vi "Colores_c.vi"() -> ()   [LabVIEW 2017]
panel:
  out "Verde 3":u32[](array[colorbox])
  out "Verde 2":u32[](array[colorbox])
  out "Azul":u32[](array[colorbox])
  out "Verde":u32[](array[colorbox])
  out "Rojo":u32[](array[colorbox])
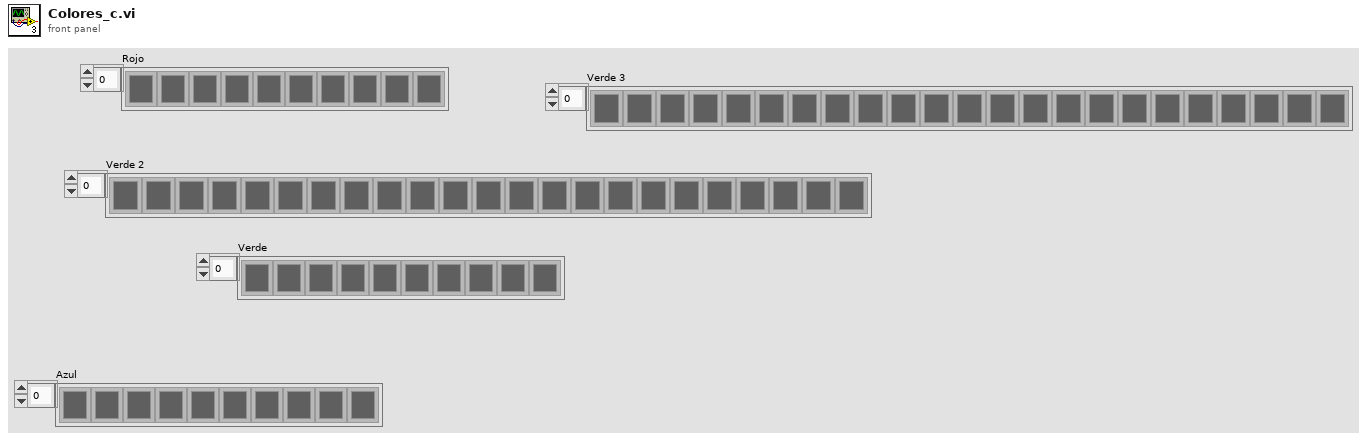
[diagram p1: front panel]
types:
  T1 = typedef "Semaphore RefNum" = refnum<k1>
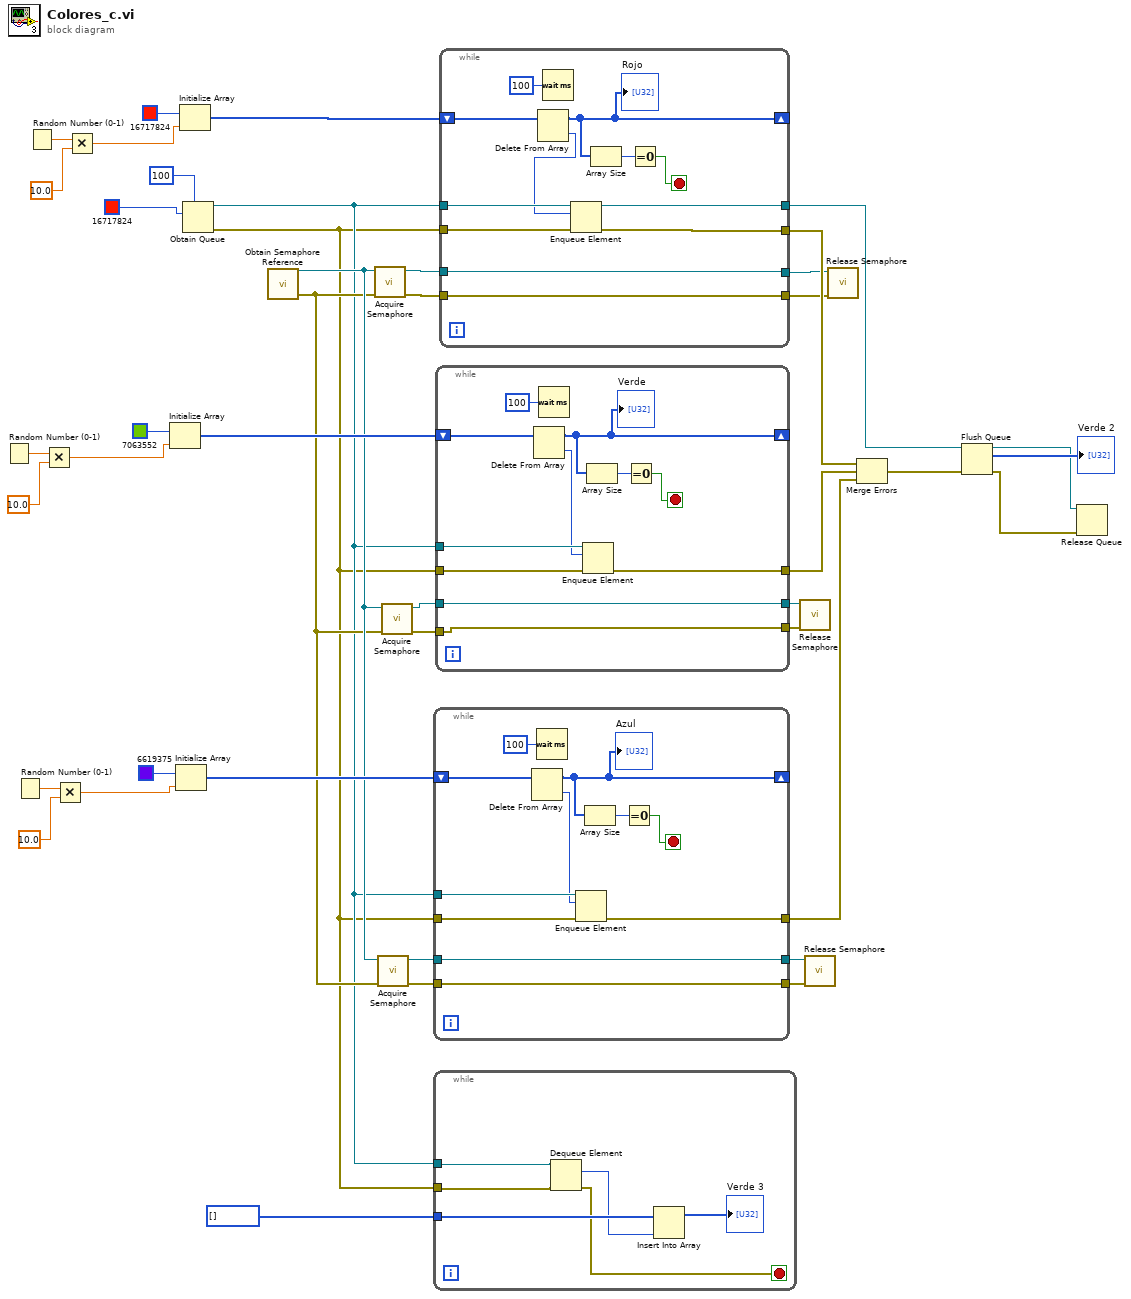
[diagram p0: block diagram]
diagram:
  n1 = Random Number (0-1)() -> (number: 0 to 1=w40:dbl)
  n2 = Random Number (0-1)() -> (number: 0 to 1=w38:dbl)
  n3 = Random Number (0-1)() -> (number: 0 to 1=w42:dbl)
  n4 = Multiply(x=w40, y=10.0) -> (x*y=w32:dbl)
  n5 = Multiply(x=w38, y=10.0) -> (x*y=w33:dbl)
  n6 = Multiply(x=w42, y=10.0) -> (x*y=w31:dbl)
  n7 = Initialize Array "Initialize Array"(u32 7063552, w32) -> (w28:u32[])
  n8 = Initialize Array "Initialize Array"(u32 6619375, w33) -> (w29:u32[])
  n9 = Initialize Array "Initialize Array"(u32 16717824, w31) -> (w30:u32[])
  n10 = Obtain Queue(max queue size (-1, unlimited)=100, element data type=u32 16717824) -> (queue out=w6:refnum<queue>, error out=w5:errorcluster)  [unwired: 3 in, 1 out]
  n11 = call <vilib>:"Obtain Semaphore Reference.vi"() -> ("error out"=w15:errorcluster, "semaphore"=w16:T1)  [unwired: 5 in, 1 out]
  n12 = call <vilib>:"Acquire Semaphore.vi"("error in (no error)"=w15, "semaphore"=w16) -> ("error out"=w18:errorcluster, "semaphore out"=w19:T1)  [unwired: 3 in, 1 out]
  n13 = call <vilib>:"Acquire Semaphore.vi"("error in (no error)"=w15, "semaphore"=w16) -> ("error out"=w12:errorcluster, "semaphore out"=w14:T1)  [unwired: 3 in, 1 out]
  n14 = call <vilib>:"Acquire Semaphore.vi"("error in (no error)"=w15, "semaphore"=w16) -> ("error out"=w10:errorcluster, "semaphore out"=w7:T1)  [unwired: 3 in, 1 out]
  n15 = while {
    shift-right: [w50] -> _
    shift-left: w29 -> [w53]
    tunnel: w6 -> [w48]
    tunnel: w5 -> [w47]
    tunnel: [w46] -> w23
    tunnel: w14 -> [w44]
    tunnel: [w44] -> w13
    tunnel: w12 -> [w43]
    tunnel: [w43] -> w11
    stop <- w51 stop-if-true
    n16 = Delete From Array(array=w53) -> (deleted portion=w45:u32, array with subset deleted=w50:u32[])  [unwired: 2 in]
    "Azul" <- w50
    n17 = Wait (ms)(milliseconds to wait=u32 100) -> ()  [unwired: 1 out]
    n18 = Enqueue Element(queue=w48, element=w45, error in (no error)=w47) -> (error out=w46:errorcluster)  [unwired: 1 in, 2 out]
    n19 = Array Size(array=w50) -> (size(s)=w52:i32)
    n20 = Equal To 0?(x=w52) -> (x = 0?=w51:bool)
  }
  n21 = while {
    tunnel: w6 -> [w58]
    tunnel: w5 -> [w57]
    tunnel: u32[] [] -> [w59]
    stop <- w56 stop-if-true
    n22 = Dequeue Element(queue=w58, error in (no error)=w57) -> (element=w55:u32, error out=w56:errorcluster)  [unwired: 1 in, 2 out]
    n23 = Insert Into Array(array=w59, new element=w55) -> (→"Verde 3":u32[])  [unwired: 1 in]
  }
  n24 = while {
    shift-right: [w67] -> _
    shift-left: w28 -> [w70]
    tunnel: w6 -> [w65]
    tunnel: w5 -> [w64]
    tunnel: [w63] -> w24
    tunnel: w10 -> [w61]
    tunnel: [w61] -> w9
    tunnel: [w60] -> w8
    tunnel: w7 -> [w60]
    stop <- w68 stop-if-true
    n25 = Delete From Array(array=w70) -> (deleted portion=w62:u32, array with subset deleted=w67:u32[])  [unwired: 2 in]
    "Verde" <- w67
    n26 = Wait (ms)(milliseconds to wait=u32 100) -> ()  [unwired: 1 out]
    n27 = Enqueue Element(queue=w65, element=w62, error in (no error)=w64) -> (error out=w63:errorcluster)  [unwired: 1 in, 2 out]
    n28 = Array Size(array=w67) -> (size(s)=w69:i32)
    n29 = Equal To 0?(x=w69) -> (x = 0?=w68:bool)
  }
  n30 = while {
    shift-right: [w79] -> _
    shift-left: w30 -> [w82]
    tunnel: w6 -> [w77]
    tunnel: w5 -> [w75]
    tunnel: [w74] -> w25
    tunnel: [w73] -> w22
    tunnel: [w72] -> w20
    tunnel: w19 -> [w72]
    tunnel: w18 -> [w71]
    tunnel: [w71] -> w17
    stop <- w80 stop-if-true
    n31 = Delete From Array(array=w82) -> (deleted portion=w76:u32, array with subset deleted=w79:u32[])  [unwired: 2 in]
    "Rojo" <- w79
    n32 = Wait (ms)(milliseconds to wait=u32 100) -> ()  [unwired: 1 out]
    n33 = Enqueue Element(queue=w77, element=w76, error in (no error)=w75) -> (queue out=w73:refnum<queue>, error out=w74:errorcluster)  [unwired: 1 in, 1 out]
    n34 = Array Size(array=w79) -> (size(s)=w81:i32)
    n35 = Equal To 0?(x=w81) -> (x = 0?=w80:bool)
  }
  n36 = call <vilib>:"Release Semaphore.vi"("error in (no error)"=w9, "semaphore"=w8) -> ()  [unwired: 4 in, 2 out]
  n37 = call <vilib>:"Release Semaphore.vi"("error in (no error)"=w11, "semaphore"=w13) -> ()  [unwired: 4 in, 2 out]
  n38 = call <vilib>:"Release Semaphore.vi"("error in (no error)"=w17, "semaphore"=w20) -> ()  [unwired: 4 in, 2 out]
  n39 = Merge Errors(w25, w24, w23) -> (w4:errorcluster)
  n40 = Flush Queue(queue=w22, error in (no error)=w4) -> (queue out=w2:refnum<queue>, remaining elements=→"Verde 2":u32[], error out=w1:errorcluster)
  n41 = Release Queue(queue=w2, error in (no error)=w1) -> ()  [unwired: 1 in, 3 out]
